vi "Untitled 3.vi"(8 "error in (no error)":errorcluster, 10 "Delay Time (s)":dbl=0.05) -> (0 "error out":errorcluster)   [LabVIEW 2016]
doc: "Inserts a time delay into the calling VI.\n--------------------\n\nThis Express VI is configured as follows:\n\nDelay Time: 0,05 s"
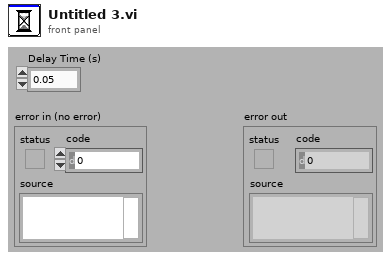
[diagram p1: front panel]
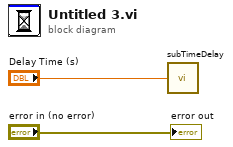
[diagram p0: block diagram]
diagram:
  n1 = call <vilib>:"subTimeDelay.vi"("Delay Time (Seconds)"="Delay Time (s)") -> ()
  "error out" <- "error in (no error)"
